vi "AutomaticExecution.vi"(7 "Measuring Limb":string, 8 "error in (no error)":errorcluster, 10 "Automatic Queue":refnum<queue>, 11 "Control.Queue":refnum<queue>) -> (0 "error out":errorcluster, 2 "Automatic Queue out":refnum<queue>)   [LabVIEW 2013, in "main.lvlib"]
uses:
  main.lvlib
panel:
  out "DisplayStr":string
  in  "Stop":bool
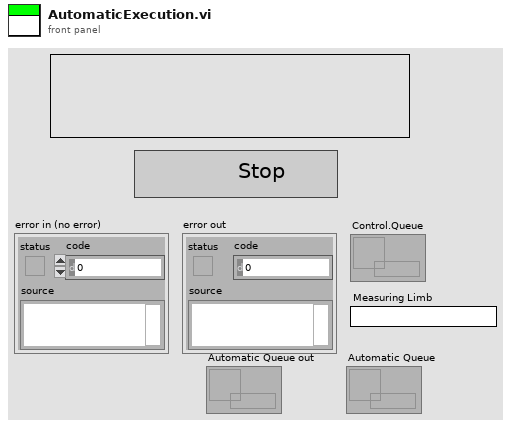
[diagram p1: front panel]
types:
  T1 = cluster{"Pump":bool, "Finger":bool, "Ankle":bool, "Fast Def":bool, "Slow Def":bool, "Init Cal":bool, "Table Pres":bool, "Table":bool}
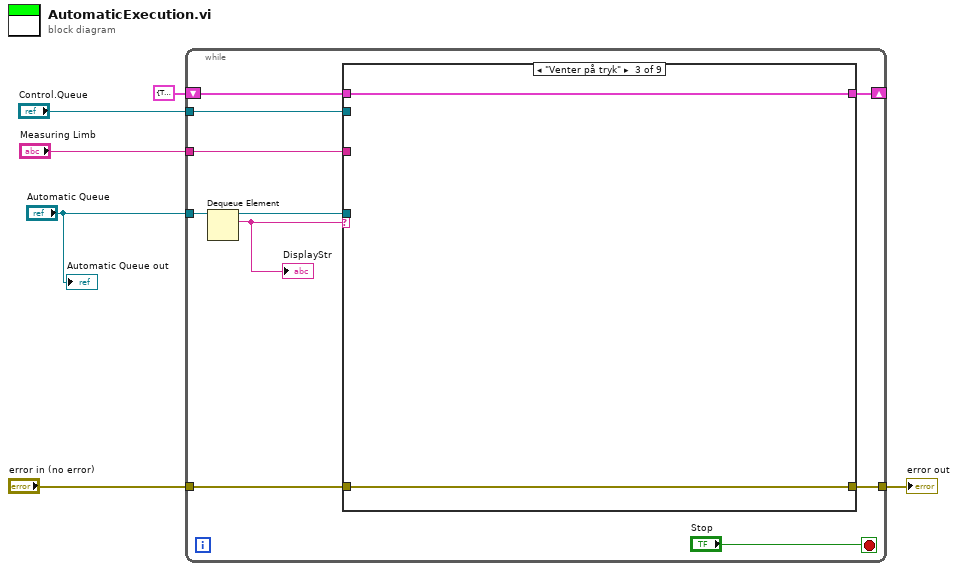
[diagram p0: block diagram]
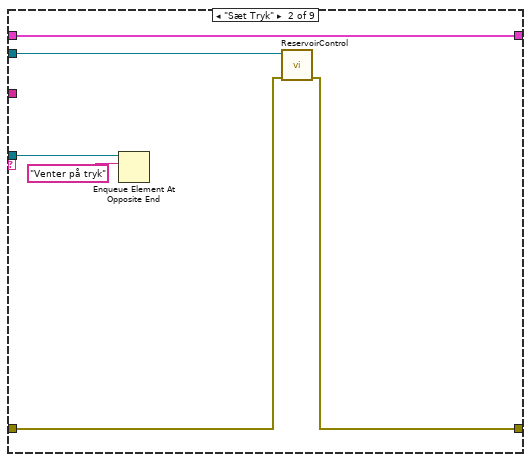
[diagram p3: hidden frame]
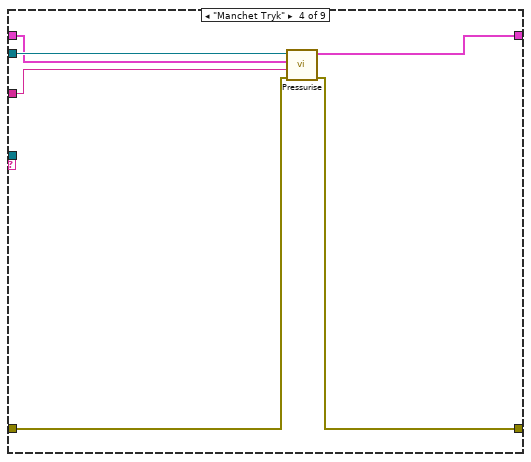
[diagram p4: hidden frame]
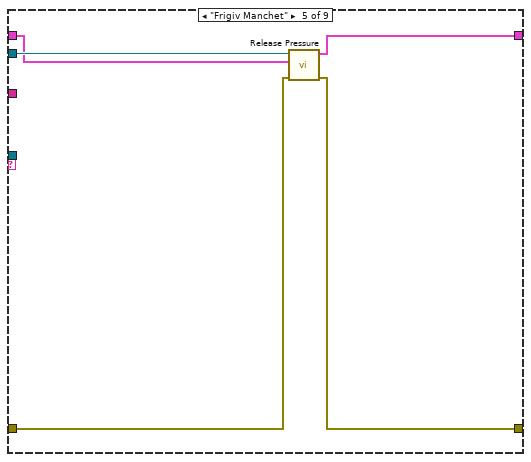
[diagram p5: hidden frame]
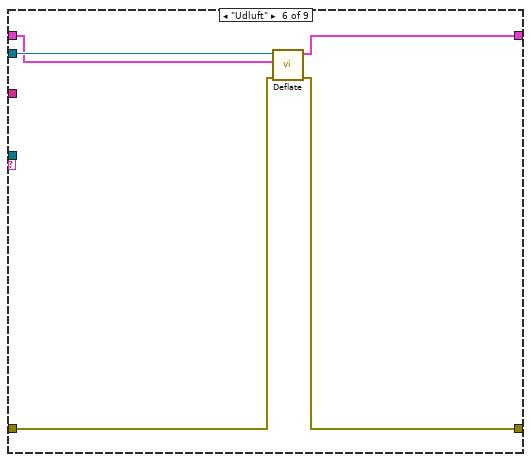
[diagram p6: hidden frame]
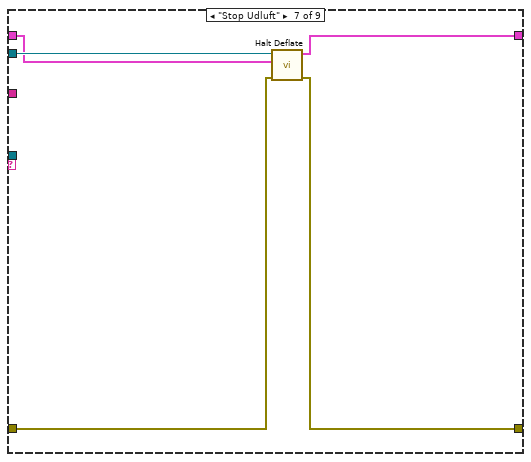
[diagram p7: hidden frame]
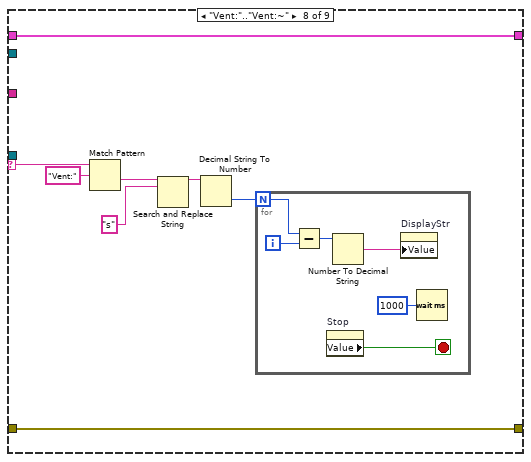
[diagram p8: hidden frame]
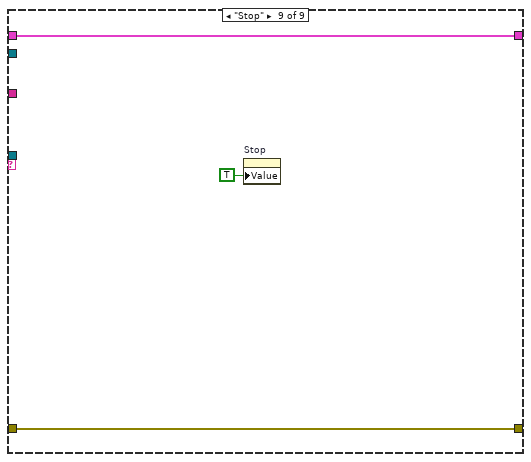
[diagram p9: hidden frame]
diagram:
  n1 = while {
    tunnel: "Automatic Queue" -> [w9]
    tunnel: "Control.Queue" -> [w15]
    tunnel: "error in (no error)" -> [w14]
    tunnel: [w13] -> w4
    shift-right: [w12] -> _
    shift-left: T1 {"Pump"=TRUE, "Finger"=TRUE, "Ankle"=TRUE, "Fast Def"=TRUE, "Slow Def"=TRUE, "Init Cal"=TRUE, "Table Pres"=TRUE, "Table"=TRUE} ("SignalCluster in") -> [w11]
    tunnel: "Measuring Limb" -> [w10]
    stop <- "Stop" stop-if-true
    n2 = Dequeue Element(queue=w9) -> (queue out=w7:refnum<queue>, element=w8:string)  [unwired: 2 in, 2 out]
    "DisplayStr" <- w8
    n3 = case shown="\"Venter på tryk\"" w8 {
      selector: w8 -> [_ _ _ _ _ _ _ w55 _]
      tunnel: w15 -> [_ w24 _ w32 w37 w42 w47 _ _]
      tunnel: w14 -> [w18 w23 w26 w31 w36 w40 w46 w50 w62]
      tunnel: [w18 w22 w26 w30 w35 w41 w45 w50 w62] -> w13
      tunnel: [w17 w21 w25 w29 w34 w39 w44 w49 w63] -> w12
      tunnel: w11 -> [w17 w21 w25 w28 w33 w38 w43 w49 w63]
      tunnel: w10 -> [_ _ _ w27 _ _ _ _ _]
      tunnel: w7 -> [_ w20 _ _ _ _ _ _ _]
      frame "", Default {
      }
      frame "Sæt Tryk" {
        n4 = Enqueue Element At Opposite End(queue=w20, element="Venter på tryk") -> ()  [unwired: 2 in, 3 out]
        n5 = call "ReservoirControl.vi"("error in (no error)"=w23, "Queue in"=w24) -> ("error out"=w22:errorcluster)  [unwired: 9 in]
      }
      frame "Venter på tryk" {
      }
      frame "Manchet Tryk" {
        n6 = call "Pressurise.vi"("error in (no error)"=w31, "Measuring Limb"=w27, "SignalCluster in"=w28, "Queue in"=w32) -> ("error out"=w30:errorcluster, "SignalCluster out"=w29:T1)  [unwired: 6 in]
      }
      frame "Frigiv Manchet" {
        n7 = call "Release Pressure.vi"("error in (no error)"=w36, "SignalCluster in"=w33, "Queue in"=w37) -> ("error out"=w35:errorcluster, "SignalCluster out"=w34:T1)  [unwired: 7 in]
      }
      frame "Udluft" {
        n8 = call "Deflate.vi"("error in (no error)"=w40, "SignalCluster in"=w38, "Queue in"=w42) -> ("error out"=w41:errorcluster, "SignalCluster out"=w39:T1)  [unwired: 7 in]
      }
      frame "Stop Udluft" {
        n9 = call "Halt Deflate.vi"("error in (no error)"=w46, "SignalCluster in"=w43, "Queue in"=w47) -> ("error out"=w45:errorcluster, "SignalCluster out"=w44:T1)  [unwired: 7 in]
      }
      frame "Vent:".."Vent:~" {
        n10 = Match Pattern(string=w55, regular expression="Vent:") -> (after substring=w52:string)  [unwired: 1 in, 3 out]
        n11 = Search and Replace String(input string=w52, search string="s") -> (result string=w53:string)  [unwired: 6 in, 3 out]
        n12 = Decimal String To Number(string=w53) -> (number=w48:i32)  [unwired: 2 in, 1 out]
        n13 = for {
          N: w48 -> [w60]
          i -> [w59]
          stop <- w56 stop-if-true
          n14 = Subtract(x=w60, y=w59) -> (x-y=w58:i32)
          n15 = property on="Stop" class="Bool (strict)"() -> ("Value"=w56:bool)  [unwired: 2 in, 2 out]
          n16 = Number To Decimal String(number=w58) -> (decimal integer string=w57:string)  [unwired: 1 in]
          n17 = property on="DisplayStr" class="Str"("Value"=w57) -> ()  [unwired: 2 in, 2 out]
          n18 = Wait (ms)(milliseconds to wait=1000 ("y")) -> ()  [unwired: 1 out]
        }
      }
      frame "Stop" {
        n19 = property on="Stop" class="Bool (strict)"("Value"=TRUE ("Stop")) -> ()  [unwired: 2 in, 2 out]
      }
    }
  }
  "error out" <- w4
  "Automatic Queue out" <- "Automatic Queue"
